vi "UnoLoopbackTesterv5.vi"() -> ()   [LabVIEW 2009]
uses:
  <vilib>/Instr/_visa.llb/VISA Configure Serial Port (Instr).vi
panel:
  in  "stop":bool
  in  "System":enum32{"Main", "Serial Terminal"}(tab)=enum."Serial Terminal"
  out "Outgoing Messages":string
  in  "Send":bool
  in  "Input":string
  out "Incoming Messages":string
  in  "VISA resource name":refnum<visa-resource-name>
  in  "baud rate (9600)":u32=9600
  in  "data bits (8)":u16=8 min=5 max=8 step=1
  in  "parity (0:none)":enum16{"None", "Odd", "Even", "Mark", "Space"}(ring)
  in  "stop bits (10: 1 bit)":u16(ring)=10 items=["1.0"=10, "1.5"=15, "2.0"=20]
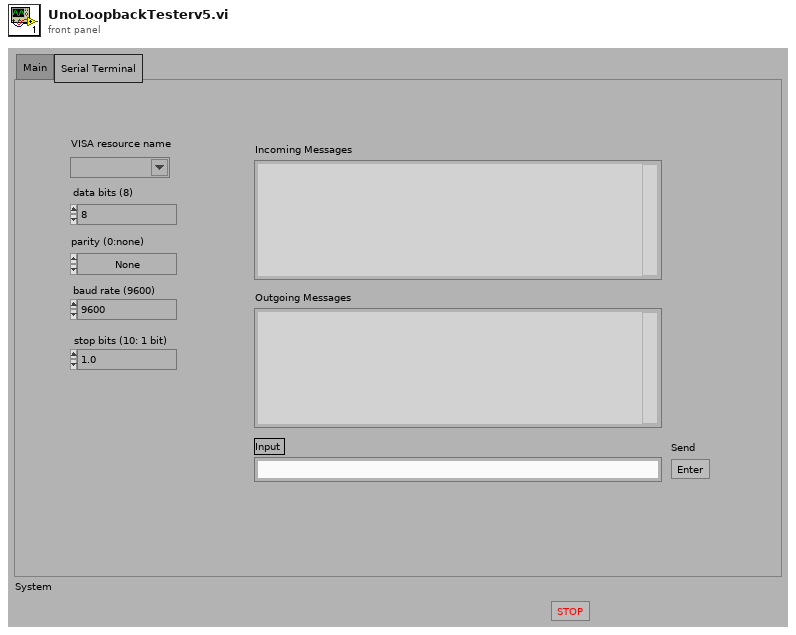
[diagram p1: front panel]
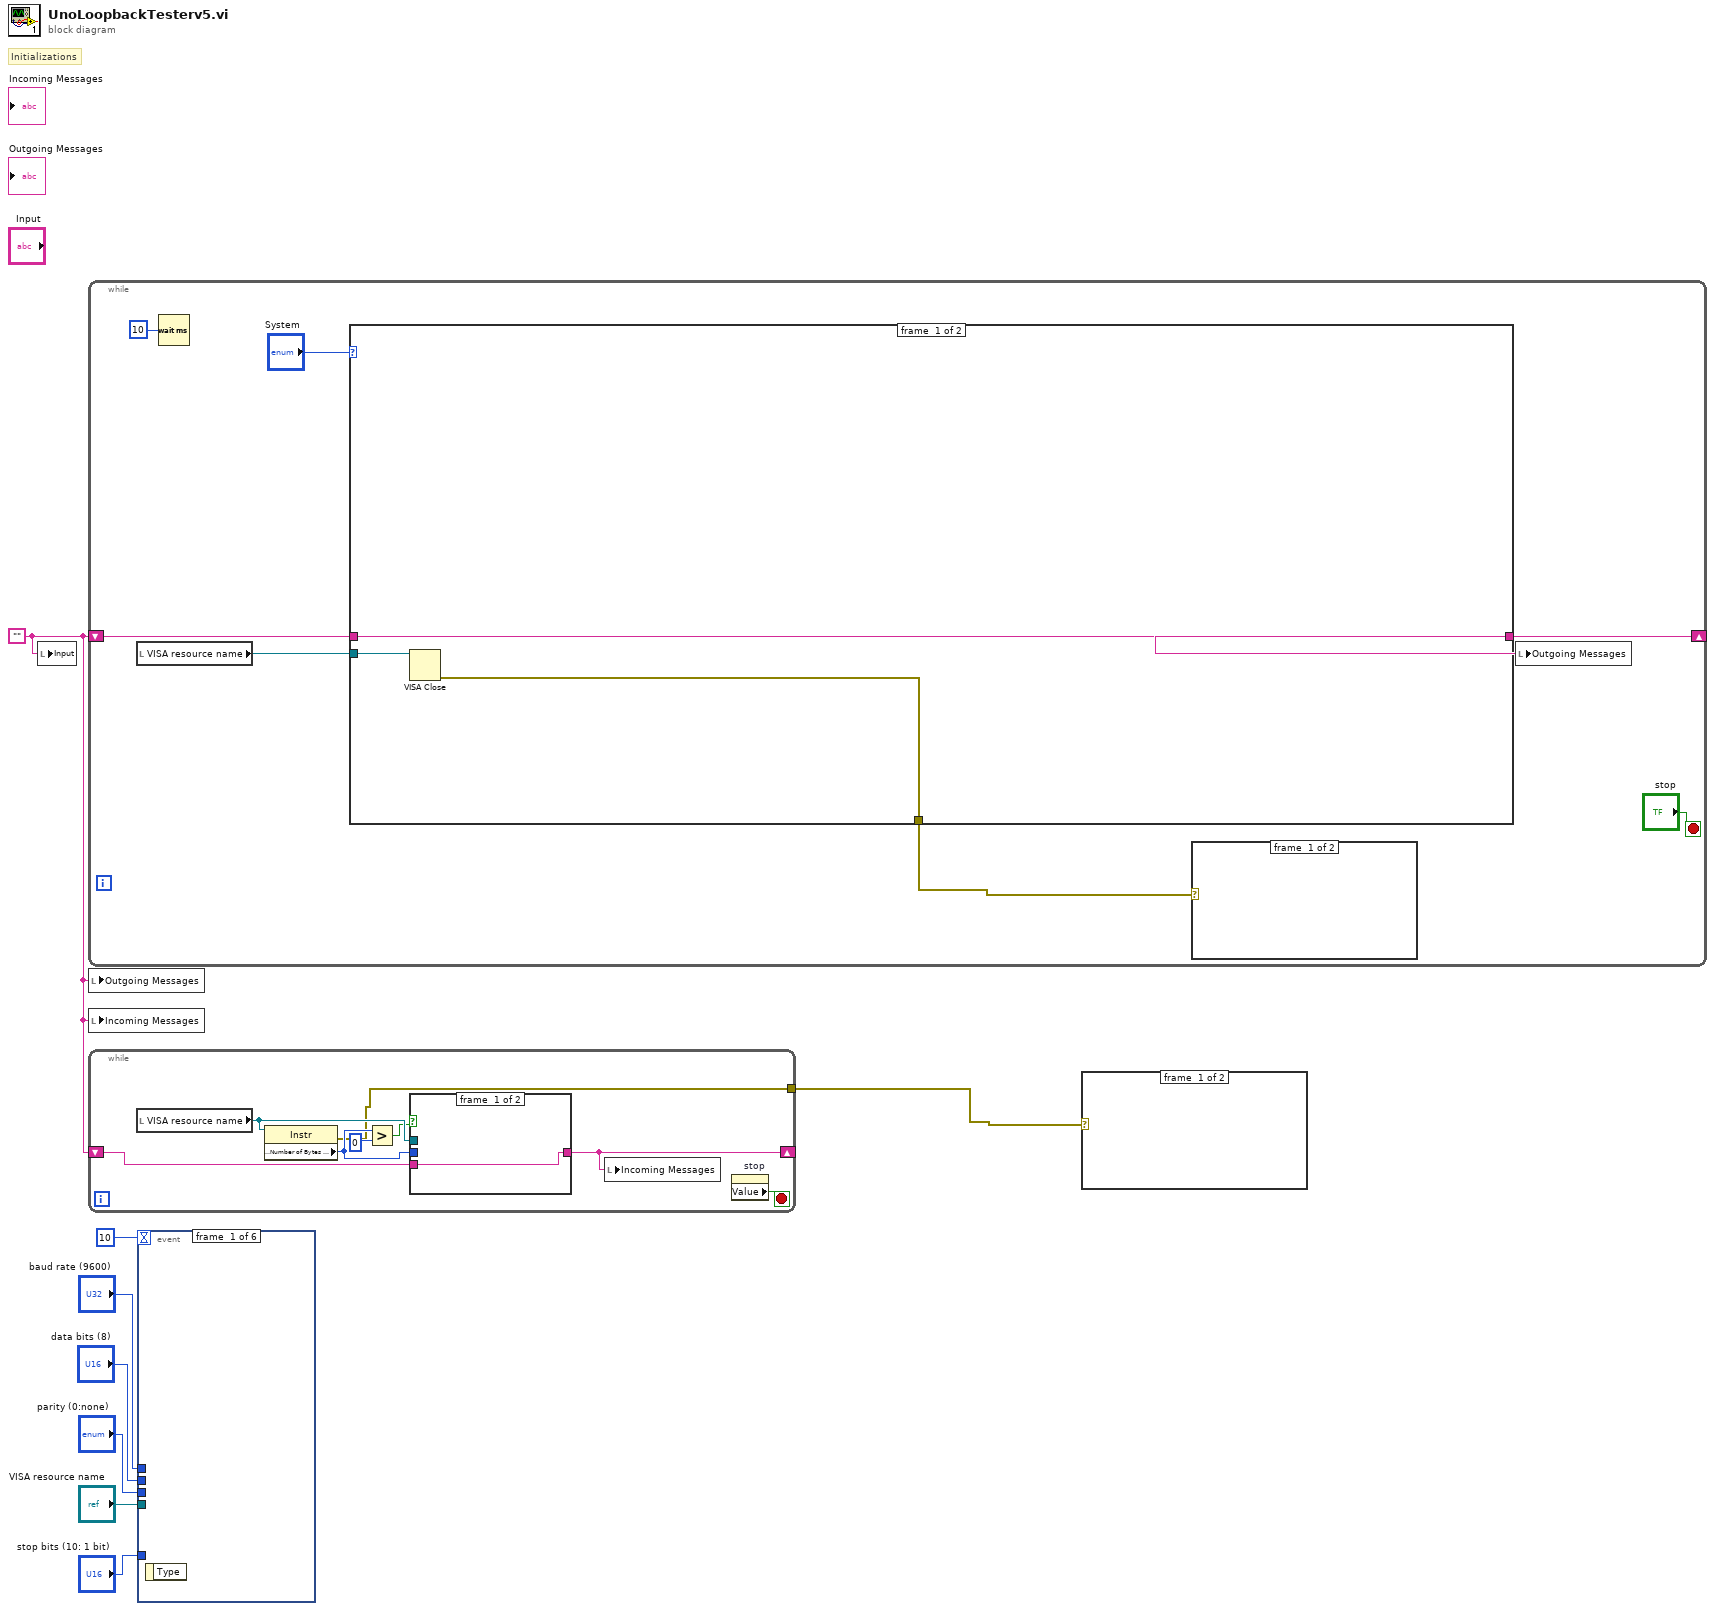
[diagram p0: block diagram]
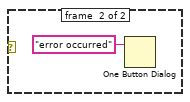
[diagram p2: hidden frame]
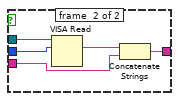
[diagram p3: hidden frame]
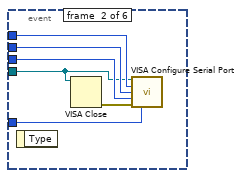
[diagram p4: hidden frame]
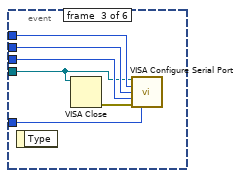
[diagram p5: hidden frame]
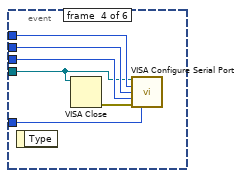
[diagram p6: hidden frame]
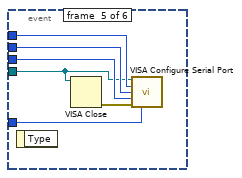
[diagram p7: hidden frame]
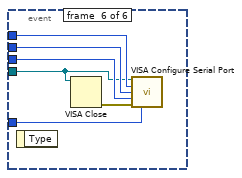
[diagram p8: hidden frame]
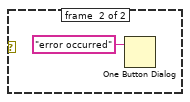
[diagram p9: hidden frame]
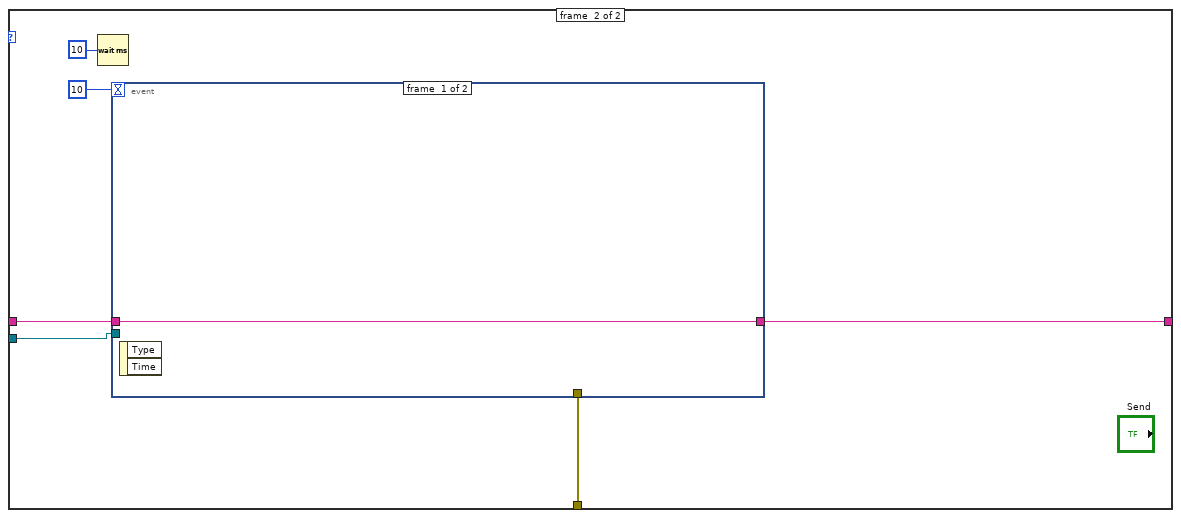
[diagram p10: hidden frame]
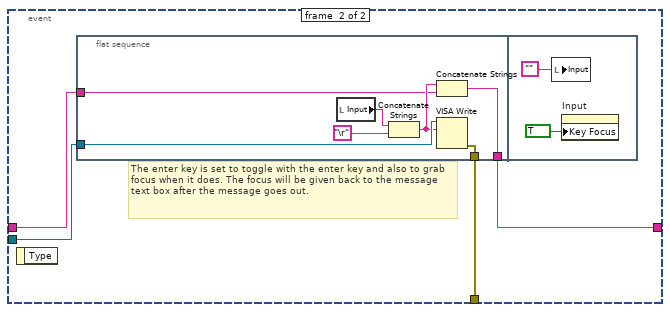
[diagram p11: hidden frame]
diagram:
  w2 = ""
  # "Initializations"
  n1 = local write "Input"(w2) -> ()
  n2 = while {
    shift-right: [w11] -> _
    shift-left: w2 -> [w12]
    stop <- "stop" stop-if-true
    n3 = local read "VISA resource name"() -> (w13:refnum<visa-resource-name>)
    n4 = Wait (ms)(milliseconds to wait=u32 10) -> ()  [unwired: 1 out]
    n5 = case shown="\"Serial Terminal\"" "System" {
      tunnel: w13 -> [w19 w23]
      tunnel: [w18 w22] -> w11
      tunnel: w12 -> [w18 w21]
      tunnel: [w17 w20] -> w9
      frame #0 {
        n6 = VISA Close(VISA resource name=w19) -> (error out=w17:errorcluster)  [unwired: 1 in]
      }
      frame #1 {
        n7 = Wait (ms)(milliseconds to wait=u32 10) -> ()  [unwired: 1 out]
        n8 = event shown="[1] \"Send\": Value Change" {
          selector: _ -> [_ _]
          dyn-events: _ -> [_ _]
          timeout: 10 -> [_ _]
          tunnel: w23 -> [_ w30]
          tunnel: [w26 w28] -> w22
          tunnel: w21 -> [w26 w29]
          tunnel: [_ w27] -> w20
          event #0 {
            n9 = event-data() -> ()  [unwired: 1 in, 2 out]
          }
          event #1 {
            # "The enter key is set to toggle with the enter key and also to grab focus when it does. The focus will be given back to the message text box after the message goes out."
            n10 = event-data() -> ()  [unwired: 1 in, 1 out]
            n11 = flat-sequence {
              tunnel: w30 -> [w35]
              tunnel: w29 -> [w33]
              tunnel: [w32] -> w28
              tunnel: [w31] -> w27
              frame #0 {
                n12 = local read "Input"() -> (w37:string)
                n13 = Concatenate Strings(w37, "\r") -> (w34:string)
                n14 = Concatenate Strings(w34, w33) -> (w32:string)
                n15 = VISA Write(VISA resource name=w35, write buffer=w34) -> (error out=w31:errorcluster)  [unwired: 1 in, 2 out]
              }
              frame #1 {
                n16 = local write "Input"("") -> ()
                n17 = property on="Input" class="Str"("Key Focus"=TRUE) -> ()  [unwired: 2 in, 2 out]
              }
            }
          }
        }
      }
    }
    n18 = case shown="Error" w9 {
      frame #0 {
      }
      frame #1 {
        n19 = One Button Dialog(message="error occurred") -> ()  [unwired: 1 in, 1 out]
      }
    }
    n20 = local write "Outgoing Messages"(w11) -> ()
  }
  n21 = local write "Outgoing Messages"(w2) -> ()
  n22 = local write "Incoming Messages"(w2) -> ()
  n23 = while {
    shift-right: [w41] -> _
    shift-left: w2 -> [w42]
    tunnel: [w40] -> w1
    stop <- w46 stop-if-true
    n24 = local read "VISA resource name"() -> (w47:refnum<visa-resource-name>)
    n25 = property class="Instr"(reference=w47) -> (error out=w40:errorcluster, "Serial Settings:Number of Bytes at Serial Port"=w43:u32)  [unwired: 1 in, 1 out]
    n26 = Greater?(x=w43, y=u32 0) -> (0:w44:bool)
    n27 = case shown="False" w44 {
      tunnel: w47 -> [_ w53]
      tunnel: w43 -> [_ w52]
      tunnel: w42 -> [w48 w49]
      tunnel: [w48 w50] -> w41
      frame #0 {
      }
      frame #1 {
        n28 = VISA Read(VISA resource name=w53, byte count=w52) -> (read buffer=w51:string)  [unwired: 1 in, 3 out]
        n29 = Concatenate Strings(w51, w49) -> (w50:string)
      }
    }
    n30 = local write "Incoming Messages"(w41) -> ()
    n31 = property on="stop" class="Bool (strict)"() -> ("Value"=w46:bool)  [unwired: 2 in, 2 out]
  }
  n32 = event shown="[5] \"stop bits (10: 1 bit)\": Value Change" {
    selector: _ -> [_ _ _ _ _ _]
    dyn-events: _ -> [_ _ _ _ _ _]
    timeout: 10 -> [_ _ _ _ _ _]
    tunnel: "VISA resource name" -> [_ w54 w60 w66 w72 w78]
    tunnel: "baud rate (9600)" -> [_ w59 w65 w71 w77 w83]
    tunnel: "data bits (8)" -> [_ w58 w64 w70 w76 w82]
    tunnel: "parity (0:none)" -> [_ w57 w63 w69 w75 w81]
    tunnel: "stop bits (10: 1 bit)" -> [_ w56 w62 w68 w74 w80]
    event #0 {
      n33 = event-data() -> ()  [unwired: 1 in, 1 out]
    }
    event #1 {
      n34 = event-data() -> ()  [unwired: 1 in, 1 out]
      n35 = VISA Close(VISA resource name=w54) -> (error out=w55:errorcluster)  [unwired: 1 in]
      n36 = call-poly "VISA Configure Serial Port"("VISA resource name"=w54, "baud rate (9600)"=w59, "data bits (8)"=w58, "parity (0:none)"=w57, "error in (no error)"=w55, "stop bits (10: 1 bit)"=w56) -> ()  [unwired: 8 in, 2 out]
    }
    event #2 {
      n37 = event-data() -> ()  [unwired: 1 in, 1 out]
      n38 = VISA Close(VISA resource name=w60) -> (error out=w61:errorcluster)  [unwired: 1 in]
      n39 = call-poly "VISA Configure Serial Port"("VISA resource name"=w60, "baud rate (9600)"=w65, "data bits (8)"=w64, "parity (0:none)"=w63, "error in (no error)"=w61, "stop bits (10: 1 bit)"=w62) -> ()  [unwired: 8 in, 2 out]
    }
    event #3 {
      n40 = event-data() -> ()  [unwired: 1 in, 1 out]
      n41 = VISA Close(VISA resource name=w66) -> (error out=w67:errorcluster)  [unwired: 1 in]
      n42 = call-poly "VISA Configure Serial Port"("VISA resource name"=w66, "baud rate (9600)"=w71, "data bits (8)"=w70, "parity (0:none)"=w69, "error in (no error)"=w67, "stop bits (10: 1 bit)"=w68) -> ()  [unwired: 8 in, 2 out]
    }
    event #4 {
      n43 = event-data() -> ()  [unwired: 1 in, 1 out]
      n44 = VISA Close(VISA resource name=w72) -> (error out=w73:errorcluster)  [unwired: 1 in]
      n45 = call-poly "VISA Configure Serial Port"("VISA resource name"=w72, "baud rate (9600)"=w77, "data bits (8)"=w76, "parity (0:none)"=w75, "error in (no error)"=w73, "stop bits (10: 1 bit)"=w74) -> ()  [unwired: 8 in, 2 out]
    }
    event #5 {
      n46 = event-data() -> ()  [unwired: 1 in, 1 out]
      n47 = VISA Close(VISA resource name=w78) -> (error out=w79:errorcluster)  [unwired: 1 in]
      n48 = call-poly "VISA Configure Serial Port"("VISA resource name"=w78, "baud rate (9600)"=w83, "data bits (8)"=w82, "parity (0:none)"=w81, "error in (no error)"=w79, "stop bits (10: 1 bit)"=w80) -> ()  [unwired: 8 in, 2 out]
    }
  }
  n49 = case shown="Error" w1 {
    frame #0 {
    }
    frame #1 {
      n50 = One Button Dialog(message="error occurred") -> ()  [unwired: 1 in, 1 out]
    }
  }
